vi "Find Discontinuity.vi"(10 "Single Record":i32=500, 11 "Data":i16[](array[numeric])) -> (2 "Discontinuity Detected":bool, 3 "cIndex":i32)   [LabVIEW 2018, in "eCRDS Library.lvlib" / "eCRDS.lvclass"]
doc: "Locate discontinuities in functions that are well behaved. This function will take the first number of entries specified by <b>Single Record</b> from <b>Data</b>and normalize those values to the range of 0 - 1. The function will detect the first discontinuity that exceeds the threshold value specified by the caller. The default value is 0.5."
uses:
  CRDS/Main/eCRDS.lvclass
panel:
  out "Waveform Graph":sgl[](graph)
  in  "threshold":sgl=0.8000001 min=0 max=1 format="%#_13g"
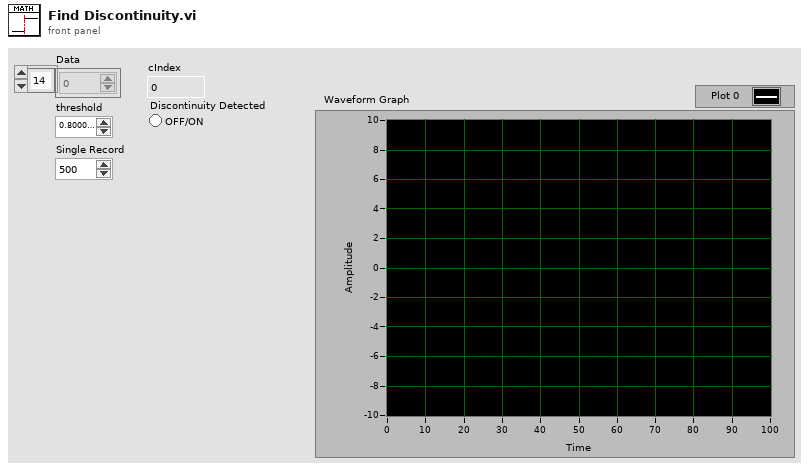
[diagram p1: front panel]
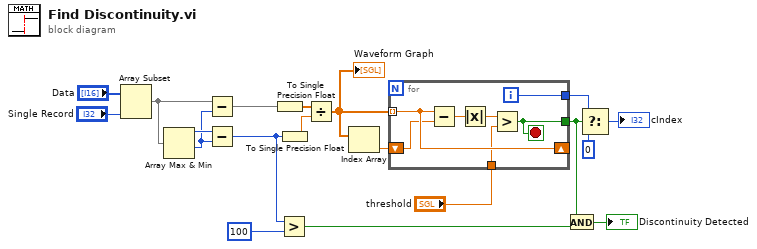
[diagram p0: block diagram]
diagram:
  n1 = Array Subset(array="Data", length="Single Record") -> (w11:i16[])  [unwired: 1 in]
  n2 = Array Max & Min(array=w11) -> (max value=w18:i16, min value=w12:i16)  [unwired: 2 out]
  n3 = Subtract(x=w11, y=w12) -> (x-y=w8:i16[])
  n4 = Subtract(x=w18, y=w12) -> (x-y=w6:i16)
  n5 = To Single Precision Float(number=w8) -> (single precision float=w9:sgl[])
  n6 = Greater?(x=w6, y=i16 100) -> (0:w3:bool)
  n7 = To Single Precision Float(number=w6) -> (single precision float=w7:sgl)
  n8 = Divide(x=w9, y=w7) -> (x/y=w1:sgl[])
  "Waveform Graph" <- w1
  n9 = Index Array(array=w1) -> (element=w13:sgl)  [unwired: 1 in]
  n10 = for {
    tunnel: w1 -> [w22] mode=indexing
    tunnel: [w24] -> w4
    tunnel: [w23] -> w16
    shift-right: [w22] -> _
    shift-left: w13 -> [w21]
    tunnel: "threshold" -> [w20]
    i -> [w23]
    stop <- w24 stop-if-true
    n11 = Subtract(x=w22, y=w21) -> (x-y=w26:sgl)
    n12 = Absolute Value(x=w26) -> (abs(x)=w25:sgl)
    n13 = Greater?(x=w25, y=w20) -> (0:w24:bool)
  }
  n14 = And(x=w4, y=w3) -> (x .and. y?=→"Discontinuity Detected":bool)
  n15 = Select(t=w16, s=w4, f=0) -> (s? t:f=→"cIndex":i32)
